vi "DistanceSensorSonarReflectionsUpdateEventExe.vi"(0 "Devices In":u64[](array[numeric]), 1 "Event Registration Refnum In":refnum<event-registration>, 5 "error in (no error)":errorcluster) -> (6 "Index":i32, 12 "Event?":bool, 13 "phid":u64, 14 "Devices Out":u64[](array[numeric]), 15 "Event Registration Refnum Out":refnum<event-registration>, 16 "Distances":u32[](array[numeric]), 17 "Amplitudes":u32[](array[numeric]), 18 "Count":u32, 19 "error out":errorcluster)   [LabVIEW 2012, in "Phidget Distance Sensor.lvlib"]
doc: "${SonarReflectionsUpdate:Header}"
uses:
  <instrlib>/Phidgets/Phidget Distance Sensor/Phidget Distance Sensor.lvlib
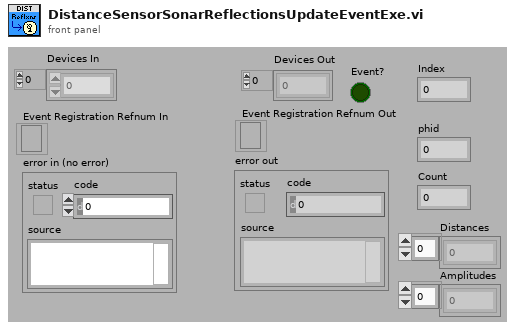
[diagram p1: front panel]
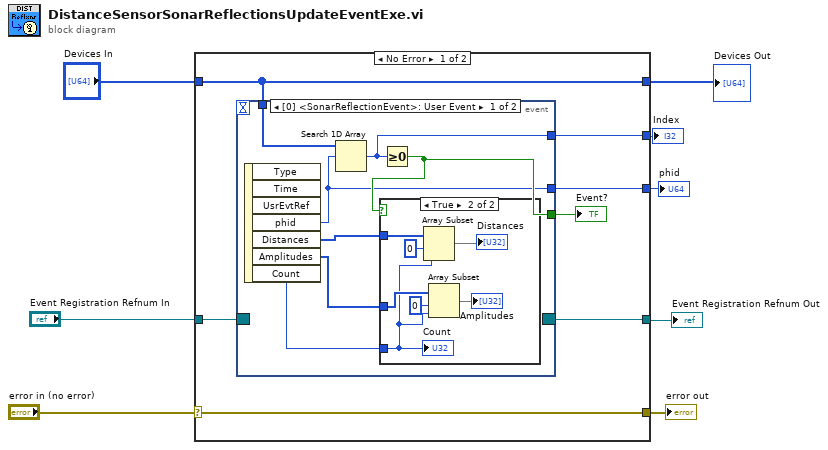
[diagram p0: block diagram]
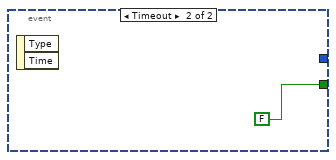
[diagram p3: hidden frame]
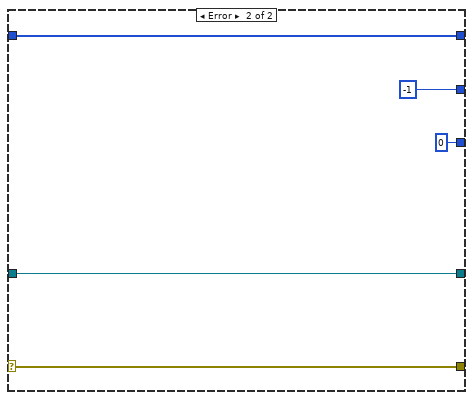
[diagram p4: hidden frame]
diagram:
  n1 = case shown="No Error" "error in (no error)" {
    selector: "error in (no error)" -> [w13 w35]
    tunnel: [w13 w35] -> w7
    tunnel: [w15 w31] -> w1
    tunnel: [w12 w34] -> w5
    tunnel: "Devices In" -> [w12 w34]
    tunnel: [w11 -1] -> w4
    tunnel: [w10 u64 0 ("phid")] -> w3
    tunnel: "Event Registration Refnum In" -> [w9 w31]
    frame No Error {
      n2 = event shown="[0] <SonarReflectionEvent>: User Event" {
        selector: w9 -> [_ _]
        dyn-events: [_ _] -> w15
        timeout: _ -> [_ _]
        tunnel: [w21 FALSE] -> w14
        tunnel: w12 -> [w22 _]
        tunnel: [w20 _] -> w11
        tunnel: [w18 _] -> w10
        event User Event {
          n3 = event-data() -> ("phid"=w18:u64, "Distances"=w19:u32[], "Amplitudes"=w17:u32[], "Count"=w16:u32)  [unwired: 1 in, 3 out]
          n4 = Search 1D Array(1D array=w22, element=w18) -> (index of element=w20:i32)  [unwired: 1 in]
          n5 = Greater Or Equal To 0?(x=w20) -> (x >= 0?=w21:bool)
          n6 = case shown="True" w21 {
            tunnel: w19 -> [_ w29]
            tunnel: w17 -> [_ w25]
            tunnel: w16 -> [_ w23]
            frame False {
            }
            frame True {
              n7 = Array Subset(array=w29, index=0, length=w23) -> (→"Distances":u32[])
              n8 = Array Subset(array=w25, index=0, length=w23) -> (→"Amplitudes":u32[])
              "Count" <- w23
            }
          }
        }
        event Timeout {
          n9 = event-data() -> ()  [unwired: 1 in, 2 out]
        }
      }
      "Event?" <- w14
    }
    frame Error {
    }
  }
  "error out" <- w7
  "Devices Out" <- w5
  "Index" <- w4
  "phid" <- w3
  "Event Registration Refnum Out" <- w1
